vi "usrednij.vi"(2 "AkcjaUsredniania":T1=enum."DodajWartość", 3 "Wartość":dbl) -> (0 "Czy kolejka pełna?":bool, 1 "Przysp. uśrednione":dbl)   [LabVIEW 2014]
uses:
  usrednijVIs/AkcjaUsredniania.ctl
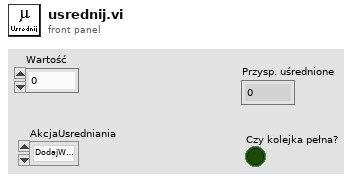
[diagram p1: front panel]
types:
  T1 = typedef "AkcjaUsredniania.ctl" = enum16{"Init", "DodajWartość", "WypełnijKolejkę", "Czyść"}
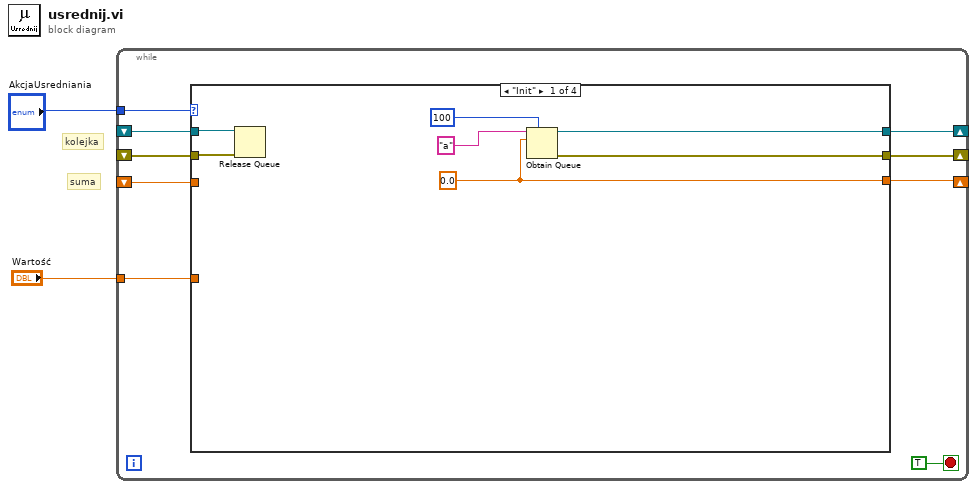
[diagram p0: block diagram]
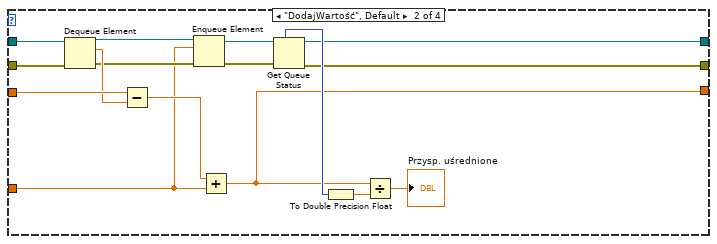
[diagram p2: hidden frame]
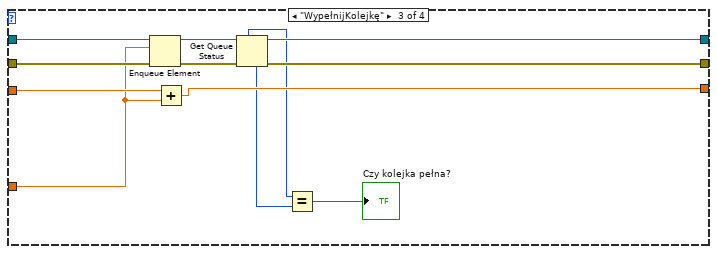
[diagram p3: hidden frame]
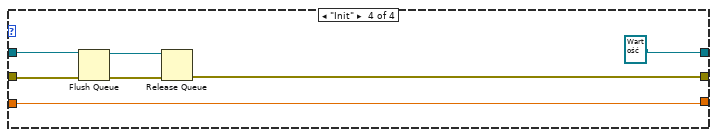
[diagram p4: hidden frame]
diagram:
  # "suma"
  # "kolejka"
  n1 = while {
    tunnel: "AkcjaUsredniania" -> [w10]
    tunnel: "Wartość" -> [w5]
    shift-right: [w9] -> _
    shift-left: _ -> [w7]
    shift-right: [w8] -> _
    shift-left: _ -> [w6]
    shift-right: [w3] -> _
    shift-left: _ -> [w4]
    stop <- TRUE stop-if-true
    n2 = case shown="\"Init\"" w10 {
      tunnel: [w17 w32 w37 refnum<queue> refnum ("queue out")] -> w9
      tunnel: [w16 w31 w38 w48] -> w8
      tunnel: w7 -> [w13 w29 w46 w53]
      tunnel: w6 -> [w12 w28 w45 w52]
      tunnel: w5 -> [_ w20 w43 _]
      tunnel: w4 -> [_ w27 w44 w47]
      tunnel: [w14 w19 w42 w47] -> w3
      frame "Init" {
        w14 = 0.0 ("Wartość")
        n3 = Release Queue(queue=w13, error in (no error)=w12) -> ()  [unwired: 1 in, 3 out]
        n4 = Obtain Queue(max queue size (-1, unlimited)=100, name (unnamed)="a", element data type=w14) -> (queue out=w17:refnum<queue>, error out=w16:errorcluster)  [unwired: 2 in, 1 out]
      }
      frame "DodajWartość", Default {
        n5 = Dequeue Element(queue=w29, error in (no error)=w28) -> (queue out=w22:refnum<queue>, element=w26:dbl, error out=w21:errorcluster)  [unwired: 1 in, 1 out]
        n6 = Subtract(x=w27, y=w26) -> (x-y=w25:dbl)
        n7 = Enqueue Element(queue=w22, element=w20, error in (no error)=w21) -> (queue out=w23:refnum<queue>, error out=w24:errorcluster)  [unwired: 1 in, 1 out]
        n8 = Add(x=w25, y=w20) -> (x+y=w19:dbl)
        n9 = Get Queue Status(queue=w23, error in (no error)=w24) -> (queue out=w32:refnum<queue>, max queue size=w33:i32, error out=w31:errorcluster)  [unwired: 1 in, 5 out]
        n10 = To Double Precision Float(number=w33) -> (double precision float=w34:dbl)
        n11 = Divide(x=w19, y=w34) -> (x/y=→"Przysp. uśrednione":dbl)
      }
      frame "WypełnijKolejkę" {
        n12 = Enqueue Element(queue=w46, element=w43, error in (no error)=w45) -> (queue out=w41:refnum<queue>, error out=w40:errorcluster)  [unwired: 1 in, 1 out]
        n13 = Add(x=w44, y=w43) -> (x+y=w42:dbl)
        n14 = Get Queue Status(queue=w41, error in (no error)=w40) -> (queue out=w37:refnum<queue>, max queue size=w35:i32, error out=w38:errorcluster, # elements in queue=w36:i32)  [unwired: 1 in, 4 out]
        n15 = Equal?(x=w35, y=w36) -> (x = y?=→"Czy kolejka pełna?":bool)
      }
      frame "Init" {
        n16 = Flush Queue(queue=w53, error in (no error)=w52) -> (queue out=w51:refnum<queue>, error out=w50:errorcluster)  [unwired: 1 out]
        n17 = Release Queue(queue=w51, error in (no error)=w50) -> (error out=w48:errorcluster)  [unwired: 1 in, 2 out]
      }
    }
  }
